vi "LUCS001RT_GPS_RS232_ReadSingleByte.vi"() -> (6 "ByteOut":u8 format="%02x")   [LabVIEW 2020]
uses:
  <vilib>/eio/EIONode/EIONode.xnode
  <vilib>/rvi/eio/common/nirviEmuTemplateMethod_errors.vi
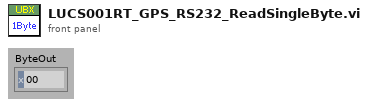
[diagram p1: front panel]
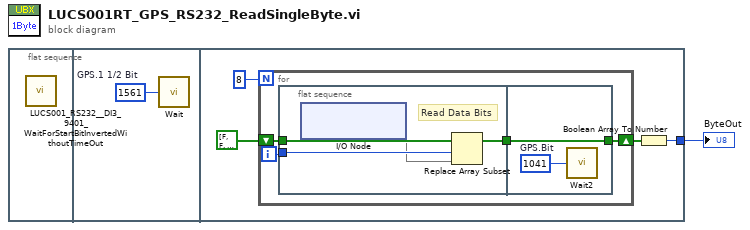
[diagram p0: block diagram]
diagram:
  n1 = flat-sequence {
    tunnel: [w3] -> w1
    frame #0 {
      n2 = call "LUCS001_RS232__DI3_9401_WaitForStartBitInvertedWithoutTimeOut.vi"() -> ()  [unwired: 12 in]
    }
    frame #1 {
      w2 = u32 1561  # GPS.1 1/2 Bit
      n3 = call "Wait"("Count(Ticks)"=w2) -> ()  [unwired: 1 out]
    }
    frame #2 {
      n4 = for {
        N: 8 ("data bits (8)") -> [_]
        shift-right: [w9] -> w5
        shift-left: bool[] [FALSE, FALSE, FALSE, FALSE, FALSE, FALSE, FALSE, FALSE] -> [w10]
        i -> [w8]
        n5 = flat-sequence {
          tunnel: w8 -> [w14]
          tunnel: w10 -> [w13]
          tunnel: [w12] -> w7
          tunnel: [w16] -> w9
          tunnel: w7 -> [w16]
          frame #0 {
            # "Read Data Bits"
            n6 = xnode "I/O Node"() -> ("Mod1/DIO3"=w11)  [unwired: 1 in, 1 out]
            n7 = Replace Array Subset(array=w13, new element=w11, index=w14) -> (w12:bool[])
          }
          frame #1 {
            w15 = u32 1041  # GPS.Bit
            n8 = call "Wait2"("Count(Ticks)"=w15) -> ()  [unwired: 1 out]
          }
        }
      }
      n9 = Boolean Array To Number(Boolean array=w5) -> (number=w3:u8)
    }
  }
  "ByteOut" <- w1
